vi "Klinger SetStatusOptions.vi"(4 "error in":errorcluster, 6 "StatusOpt":T1={"AXIS MOVING"=TRUE, "W & X TRAVEL LIMIT"=TRUE, "Y & Z TRAVEL LIMIT"=TRUE, "INPUT BITS VALUE"=TRUE, "W  POSITION"=TRUE, "X  POSITION"=TRUE, "Y  POSITION"=TRUE, "Z  POSITION"=TRUE} caption="Status Report Options", 7 "addresse":string="6") -> (0 "error out":errorcluster)   [LabVIEW 2010]
doc: "Ce VI permet de régler les options de rapport de statut du contrôleur.Celle-ci détermines les informations qui seront envoyer lors d'une lecture ou à la suite de la commande \"?\""
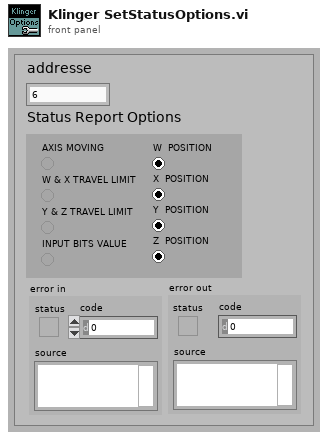
[diagram p1: front panel]
types:
  T1 = cluster{"AXIS MOVING":bool, "W & X TRAVEL LIMIT":bool, "Y & Z TRAVEL LIMIT":bool, "INPUT BITS VALUE":bool, "W  POSITION":bool, "X  POSITION":bool, "Y  POSITION":bool, "Z  POSITION":bool}
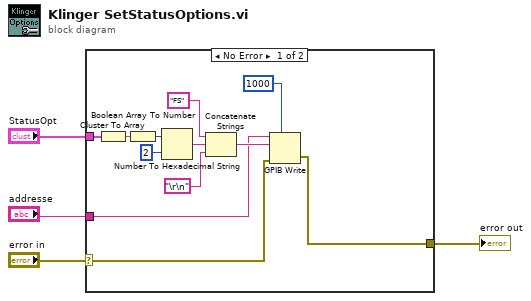
[diagram p0: block diagram]
diagram:
  n1 = case shown="No Error" "error in" {
    tunnel: [w5 w17] -> w4
    tunnel: "StatusOpt" -> [w12 _]
    tunnel: "addresse" -> [w7 _]
    selector: "error in" -> [w8 w17]
    frame No Error {
      n2 = Cluster To Array(cluster=w12) -> (array=w11:bool[])
      n3 = Boolean Array To Number(Boolean array=w11) -> (number=w10:u32)
      n4 = Number To Hexadecimal String(1:i16 2 ("width (-)"), 2:w10) -> (0:w9:string)
      n5 = Concatenate Strings("FS", w9, "\r\n") -> (w16:string)
      n6 = GPIB Write(0:w7, 1:w16, 3:w8, 4:1000 ("timeout ms (488.2 global)")) -> (6:w5:errorcluster)  [unwired: 1 in, 1 out]
    }
    frame Error {
    }
  }
  "error out" <- w4
